vi "Control setpoint.vi"(11 "Meerstetter Lib.lvlib:TEC 1090":refnum<class "Meerstetter TEC.lvclass">) -> (3 "Meerstetter Lib.lvlib:TEC 1091":refnum<class "Meerstetter TEC.lvclass">)   [LabVIEW 2014, in "Meerstetter Lib.lvlib" / "Meerstetter TEC.lvclass"]
uses:
  Meerstetter TEC.lvclass
  Meerstetter TEC.lvclass/Meerstetter TEC.ctl
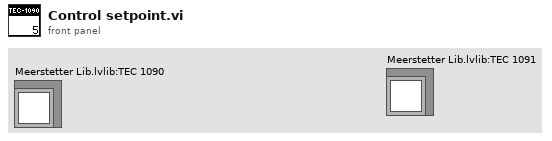
[diagram p1: front panel]
types:
  T1 = typedef "Ctl Method.ctl" = enum16{"Temperature", "Power"}
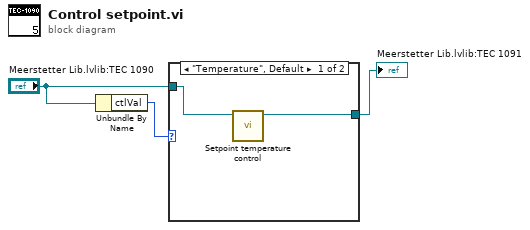
[diagram p0: block diagram]
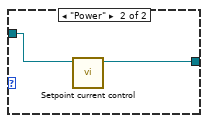
[diagram p2: hidden frame]
diagram:
  n1 = Unbundle By Name("Meerstetter Lib.lvlib:TEC 1090") -> ("ctlVal"=w3:T1)
  n2 = case shown="\"Temperature\", Default" w3 {
    tunnel: "Meerstetter Lib.lvlib:TEC 1090" -> [w5 w7]
    tunnel: [w4 w6] -> w1
    frame "Temperature", Default {
      n3 = call "Setpoint temperature control.vi"("Meerstetter Lib.lvlib:TEC 1090"=w5) -> ("TEC 1090 out"=w4:refnum<class "Meerstetter TEC.lvclass">)  [unwired: 9 in, 1 out]
    }
    frame "Power" {
      n4 = call "Setpoint current control.vi"("Meerstetter Lib.lvlib:TEC 1090"=w7) -> ("TEC 1090 out"=w6:refnum<class "Meerstetter TEC.lvclass">)  [unwired: 9 in, 1 out]
    }
  }
  "Meerstetter Lib.lvlib:TEC 1091" <- w1
